vi "Build data wavef.vi"(1 "Boolean":bool, 2 "Array 2":waveform(dbl)[](array[waveform])) -> (0 "Array":waveform(dbl)[](array[waveform]))   [LabVIEW 2020]
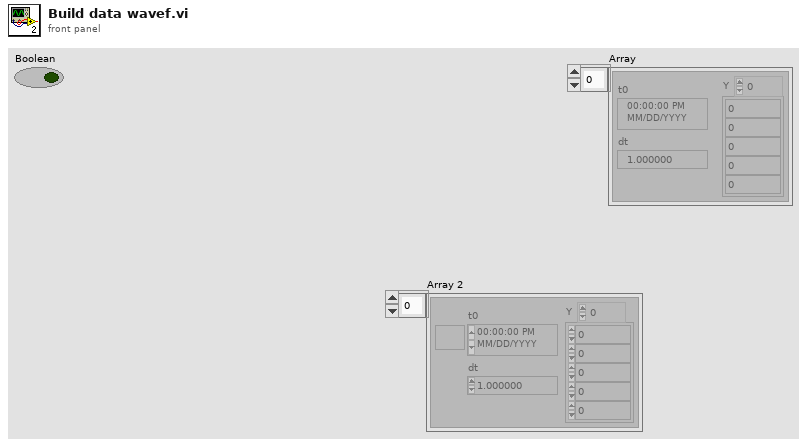
[diagram p1: front panel]
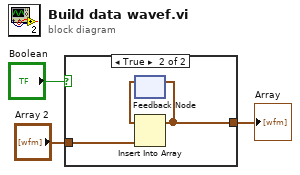
[diagram p0: block diagram]
diagram:
  n1 = case shown="True" "Boolean" {
    tunnel: "Array 2" -> [w4 w6]
    tunnel: [w4 w5] -> w2
    frame False {
    }
    frame True {
      n2 = feedback #1() -> (w7:waveform(dbl)[])  [unwired: 1 in]
      n3 = Insert Into Array(array=w7, new element=w6) -> (w5:waveform(dbl)[])  [unwired: 1 in]
      n4 = feedback-in #1(w5) -> ()
    }
  }
  "Array" <- w2
